vi "WinBYTE.vi"() -> ()   [LabVIEW 2014]
doc: "This function performs an AND of the input with 0xAA and returns the result.\n\nFor information on the data types used for the DLL function, right-click on the Call Library Function node and choose Configure."
uses:
  CLF_Example.dll
panel:
  out "output":u8 format="%08b"
  in  "input":u8=255 format="%08b"
  # "See the block diagram for more information."
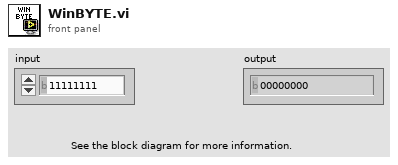
[diagram p1: front panel]
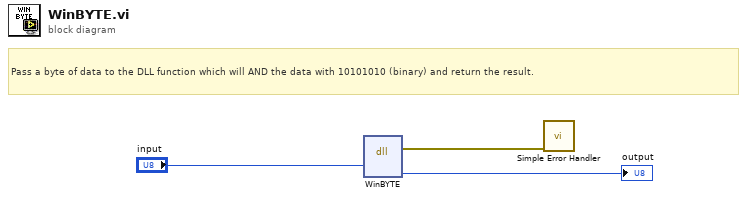
[diagram p0: block diagram]
diagram:
  # "Pass a byte of data to the DLL function which will AND the data with 10101010 (binary) and return the result."
  n1 = dll-call lib="e:/builds/penguin/labview/branches/2014/dev/dist/examples/Connectivity/Libraries and Executables/DLL Calling VIs/CLF_Example**.*" fn="WinBYTE"("input"="input") -> (error out=w1:errorcluster, "output"=→"output":u8)  [unwired: 4 in, 3 out]
  n2 = call <vilib>:"Simple Error Handler.vi"("error in (no error)"=w1) -> ()  [unwired: 4 in, 5 out]
